vi "PCO_GetColorValues.vi"(8 "error in (no error)":errorcluster {"code" format="%x"}, 9 "iBlueMax":i32, 10 "iGreenMax":i32, 11 "iRedMax":i32) -> (0 "error out":errorcluster {"code" format="%x"}, 1 "pfColorTint":sgl, 2 "pfColorTemp":sgl, 3 "ErrorMessage":i32 format="%x")   [LabVIEW 2020, in "Convert.lvlib"]
doc: "int PCOCONVERT_API PCO_GetColorValues(float *pfColorTemp, float *pfColorTint, int iRedMax, int iGreenMax, int iBlueMax);"
uses:
  Convert.lvlib
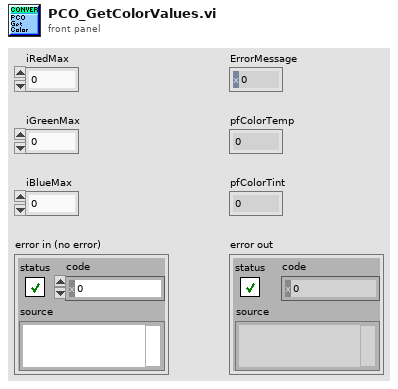
[diagram p1: front panel]
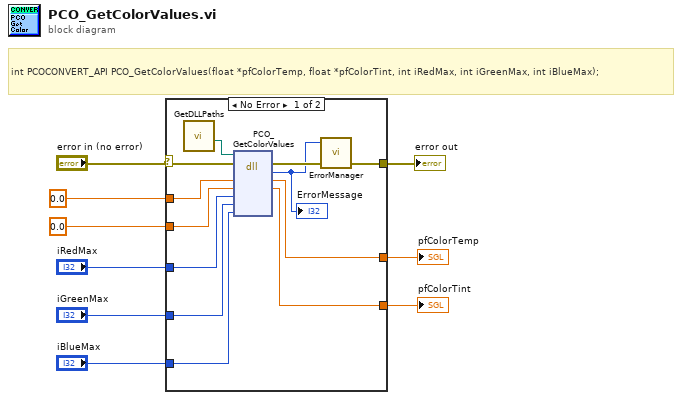
[diagram p0: block diagram]
diagram:
  # "int PCOCONVERT_API PCO_GetColorValues(float *pfColorTemp, float *pfColorTint, int iRedMax, int iGreenMax, int iBlueMax);"
  n1 = case shown="No Error" "error in (no error)" {
    selector: "error in (no error)" -> [w16 w22]
    tunnel: [w21 w24] -> w9
    tunnel: [w20 w23] -> w8
    tunnel: "iRedMax" -> [w19 _]
    tunnel: "iGreenMax" -> [w18 _]
    tunnel: "iBlueMax" -> [w17 _]
    tunnel: [w14 w22] -> w4
    tunnel: sgl 0.0 ("pfColorTemp") -> [w11 w24]
    tunnel: sgl 0.0 ("pfColorTint") -> [w12 w23]
    frame No Error {
      n2 = call "GetDLLPaths.vi"() -> ("PCO_Conv_Path"=w10:path)  [unwired: 9 in, 2 out]
      n3 = dll-call lib="?" fn="PCO_GetColorValues"(path in=w10, error in=w16, "pfColorTemp"=w11, "pfColorTint"=w12, "iRedMax"=w19, "iGreenMax"=w18, "iBlueMax"=w17) -> (error out=w15:errorcluster, "return type"=w13:i32, "pfColorTemp"=w21:sgl, "pfColorTint"=w20:sgl)  [unwired: 4 in, 1 out]
      "ErrorMessage" <- w13
      n4 = call "ErrorManager.vi"("error in (no error)"=w15, "error code"=w13) -> ("error out"=w14:errorcluster)  [unwired: 3 in]
    }
    frame Error {
    }
  }
  "pfColorTemp" <- w9
  "pfColorTint" <- w8
  "error out" <- w4
